vi "SetPos.vi"(2 "error in (no error)":errorcluster, 3 "NewPosition":dbl format="%#_13g", 4 "StepperController in":refnum<class "StepperController.lvclass">) -> (0 "error out":errorcluster, 1 "StepperController out":refnum<class "StepperController.lvclass">)   [LabVIEW 2013, in "StepperController.lvclass"]
uses:
  StepperController.lvclass
  StepperController.lvclass/StepperController.ctl
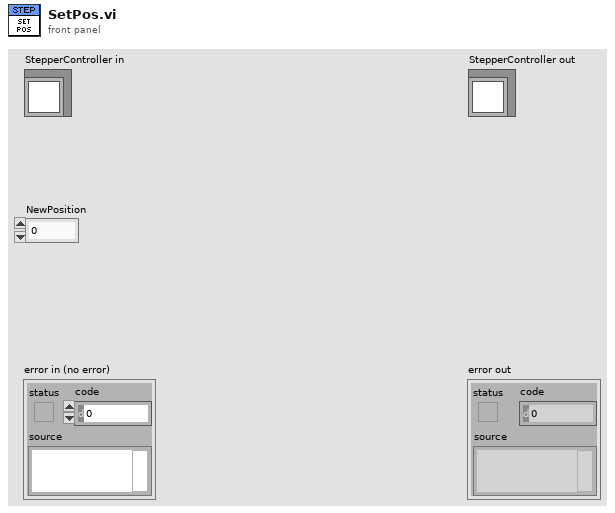
[diagram p1: front panel]
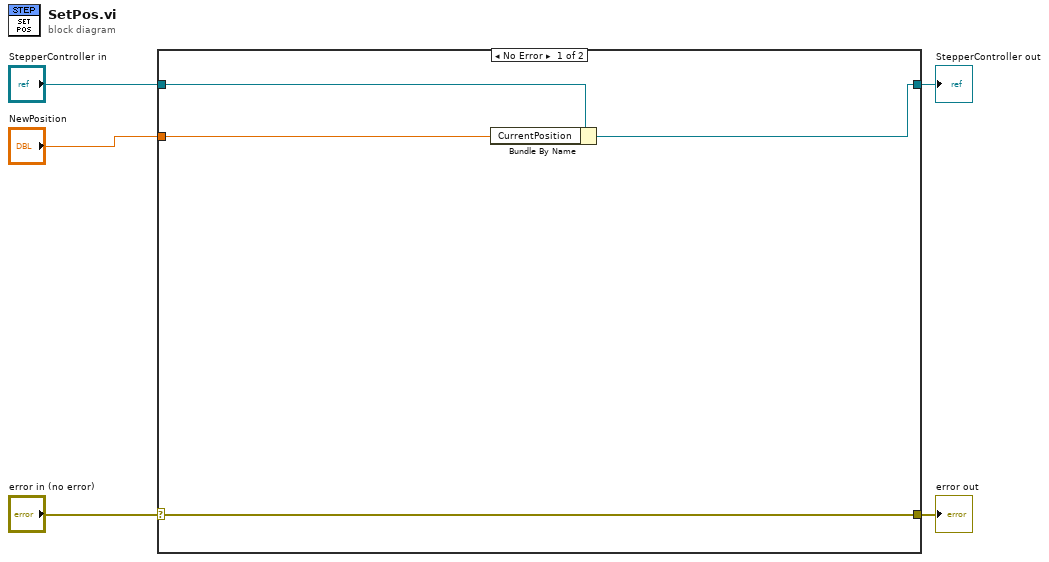
[diagram p0: block diagram]
diagram:
  n1 = case shown="No Error" "error in (no error)" {
    selector: "error in (no error)" -> [w9 w10]
    tunnel: [w9 w10] -> w4
    tunnel: [w7 w11] -> w2
    tunnel: "StepperController in" -> [w8 w11]
    tunnel: "NewPosition" -> [w6 _]
    frame No Error {
      n2 = Bundle By Name(cluster=w8, "CurrentPosition"=w6) -> (w7:refnum<class "StepperController.lvclass">)
    }
    frame Error {
    }
  }
  "error out" <- w4
  "StepperController out" <- w2
